vi "Status Moving Mono.vi"(11 "VISA resource name":refnum<visa-resource-name>="COM6") -> (1 "moving?":bool, 3 "read buffer":string)   [LabVIEW 2022 SP3]
panel:
  out "?":refnum<visa-resource-name>
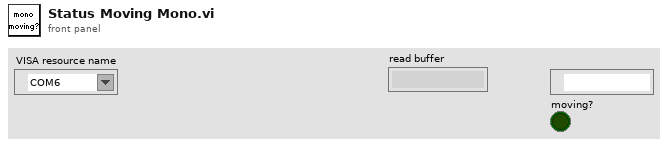
[diagram p1: front panel]
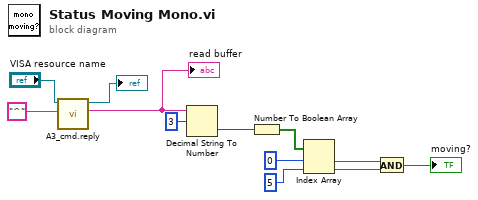
[diagram p0: block diagram]
diagram:
  n1 = call "A3_cmd.reply.vi"("cmd"="^" ("write buffer"), "VISA resource name"="VISA resource name") -> ("reply"=w12:string, "VISA resource name out"=→"?":refnum<visa-resource-name>)  [unwired: 7 in, 1 out]
  "read buffer" <- w12
  n2 = Decimal String To Number(string=w12, offset=3) -> (number=w4:i32)  [unwired: 1 in, 1 out]
  n3 = Number To Boolean Array(number=w4) -> (Boolean array=w8:bool[])
  n4 = Index Array(array=w8, index #1=0 ("index"), index #2=5 ("index")) -> (element #1=w2:bool, element #2=w3:bool)
  n5 = And(x=w2, y=w3) -> (x .and. y?=→"moving?":bool)
